vi "XYZ STAGE SERVER.vi"() -> ()   [LabVIEW 2018]
uses:
  STAGE POSITION.ctl
  GOTO POSITION.ctl
  STAGE VELOCITY.ctl
  FIB STAGE EVENTS.ctl
panel:
  in  "OBJECT RANGE":i32(ring) items=["100um", "150um", "200um", "250um", "500um ", "0-1mm Variable", "1mm Aperture", "2mm Aperture", "5mm Aperture", "OPEN"]
  out "VALID SESSION":bool=TRUE
  out "PZ":i32
  out "PY":i32
  out "PX":i32
  in  "ZERO STAGES":bool
  in  "Array":cluster{"POSITION ":T1, "MARKER ID":string}[](array[cluster]) {"POSITION"."Z" format="%_5g"; "POSITION"."Y" format="%_5g"; "POSITION"."X" format="%_5g"}
  out "REPLY":string[](array[string])
  out "COMMAND":string[](array[string])
  out "STAGE ERROR":errorcluster={"status"=FALSE, "code"=1073676293, "source"="VISA Read in ARCUS Object Socket.vi->CSIRO Object Control Ethernet.vi"}
  out "FIB STAGE":refnum<visa-resource-name>="CSIRO-OBJECT"
  out "Z":bool[](array[boolean])=[FALSE, FALSE, FALSE, FALSE, FALSE, FALSE, TRUE, FALSE, FALSE, FALSE, FALSE, FALSE, FALSE, FALSE, FALSE, FALSE]
  out "X":bool[](array[boolean])=[FALSE, FALSE, FALSE, FALSE, FALSE, FALSE, TRUE, FALSE, FALSE, FALSE, FALSE, FALSE, FALSE, FALSE, FALSE, FALSE]
  out "THETA":bool[](array[boolean])=[FALSE, FALSE, FALSE, FALSE, FALSE, FALSE, TRUE, FALSE, FALSE, FALSE, FALSE, FALSE, FALSE, FALSE, FALSE, FALSE]
  out "Y":bool[](array[boolean])=[FALSE, FALSE, FALSE, FALSE, FALSE, FALSE, TRUE, FALSE, FALSE, FALSE, FALSE, FALSE, FALSE, FALSE, FALSE, FALSE]
  in  "RIGHT":bool=TRUE
  in  "LEFT":bool=TRUE
  in  "CLEAR":bool
  out "ERROR OUT":errorcluster
  in  "Tab Control":enum32{"STAGE CONTROL", "VELOCITY/ACC/CAL"}(tab)
  out "POSITION":T1 {"Z" format="%#_5g"; "Y" format="%#_5g"; "X" format="%#_5g"}
  in  "GOTO POSITION":T2 {"Z" format="%#_4g"; "Y" min=-0.019999999552965164 max=0.019999999552965164 step=9.999999747378752e-05 format="%#_5g"; "X" format="%#_5g"}
  out "ZCAL STATUS":bool
  out "YCAL STATUS":bool
  out "XCAL STATUS":bool
  in  "HOME Z":bool
  in  "HOME Y":bool
  in  "HOME X":bool
  in  "XYZ STAGE JOG":T3={"DOWN"=FALSE, "UP"=FALSE, "STEP SIZE"=1, "LEFT"=FALSE, "RIGHT"=FALSE} {"STEP SIZE" items=["1 um", "5 um", "20 um", "50 um", "100 um", "500 um", "2000 um"]}
  in  "ABORT":bool
  in  "STOP":bool
  out "CONTROLLER IP":string="10.100.12.76"
  in  "STAGE VELOCITIES":T4={"X VEL"=0.0020000000949949026, "Y VEL"=0.0020000000949949026, "Z VEL"=0.0010000000474974513} {"X VEL" format="%_2f"}
  in  "STAGE ACCELERATION":T5={"X VEL"=0.05, "Y VEL"=0.05, "Z VEL"=0.0010000000474974513} {"X VEL" format="%_2f"}
  in  "YA":dbl[unit]=2.55e-10 format="%#_5g"
  in  "YB":dbl[unit]=0.000128 format="%#_5g"
  in  "XA":dbl[unit]=2.55e-10 format="%#_5g"
  in  "XB":dbl[unit]=0.000125 format="%#_5g"
  in  "ZA":dbl[unit]=2.55e-10 format="%#_5g"
  in  "ZB":dbl[unit]=0.000128 format="%#_5g"
  in  "OYACC":i32=300 min=1 max=5000
  in  "OXACC":i32=300 min=1 max=5000
  in  "OHSPEED":i32=20000 min=1 max=400000 step=1
  in  "OLSPEED":i32=2000 min=100 max=490550
  # "MOTOR ACCE"
  # "MOTOR DECC"
  # "CONST SPEED"
  # "IN ALARM"
  # "LIMIT+ INPUT"
  # "LIMIT- INPUT"
  # "HOME INPUT"
  # "LIMIT+ERROR"
  # "LIMIT- ERROR"
  # "ALARM ERROR"
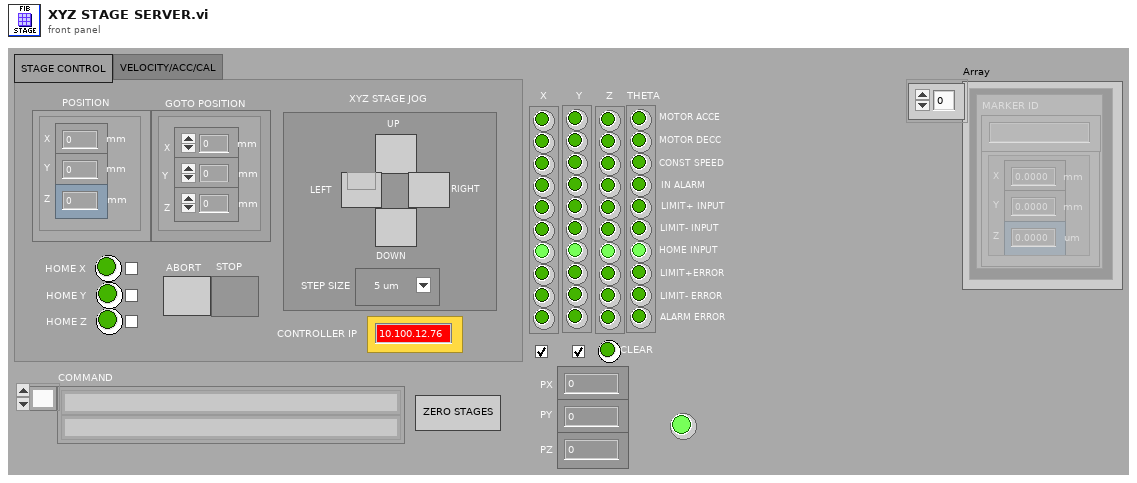
[diagram p1: front panel]
types:
  T1 = typedef "STAGE POSITION.ctl" = cluster{"X":dbl[unit], "Y":dbl[unit], "Z":dbl[unit]}
  T2 = typedef "GOTO POSITION.ctl" = cluster{"X":dbl[unit], "Y":dbl[unit], "Z":dbl[unit]}
  T3 = cluster{"DOWN":bool, "UP":bool, "STEP SIZE":u16, "LEFT":bool, "RIGHT":bool}
  T4 = typedef "STAGE VELOCITY.ctl" = cluster{"X VEL":dbl[unit], "Y VEL":dbl[unit], "Z VEL":dbl[unit]}
  T5 = cluster{"X VEL":dbl[unit], "Y VEL":dbl[unit], "Z VEL":dbl[unit]}
  T6 = typedef "FIB STAGE EVENTS.ctl" = enum16{"LOOP", "INIT STAGE CONTROLLER", "SEND COMMAND TO CONTROLLER", "HOME X", "HOME Y", "HOME Z", "ABORT ALL AXES", "GOTO MARKER", "ZERO XYZ", "READ XYZ POSITIONS", "GOTO XYZ POSITION", "STOP", "JOG XYZ", "WAIT FOR MOVE COMPLETE"}
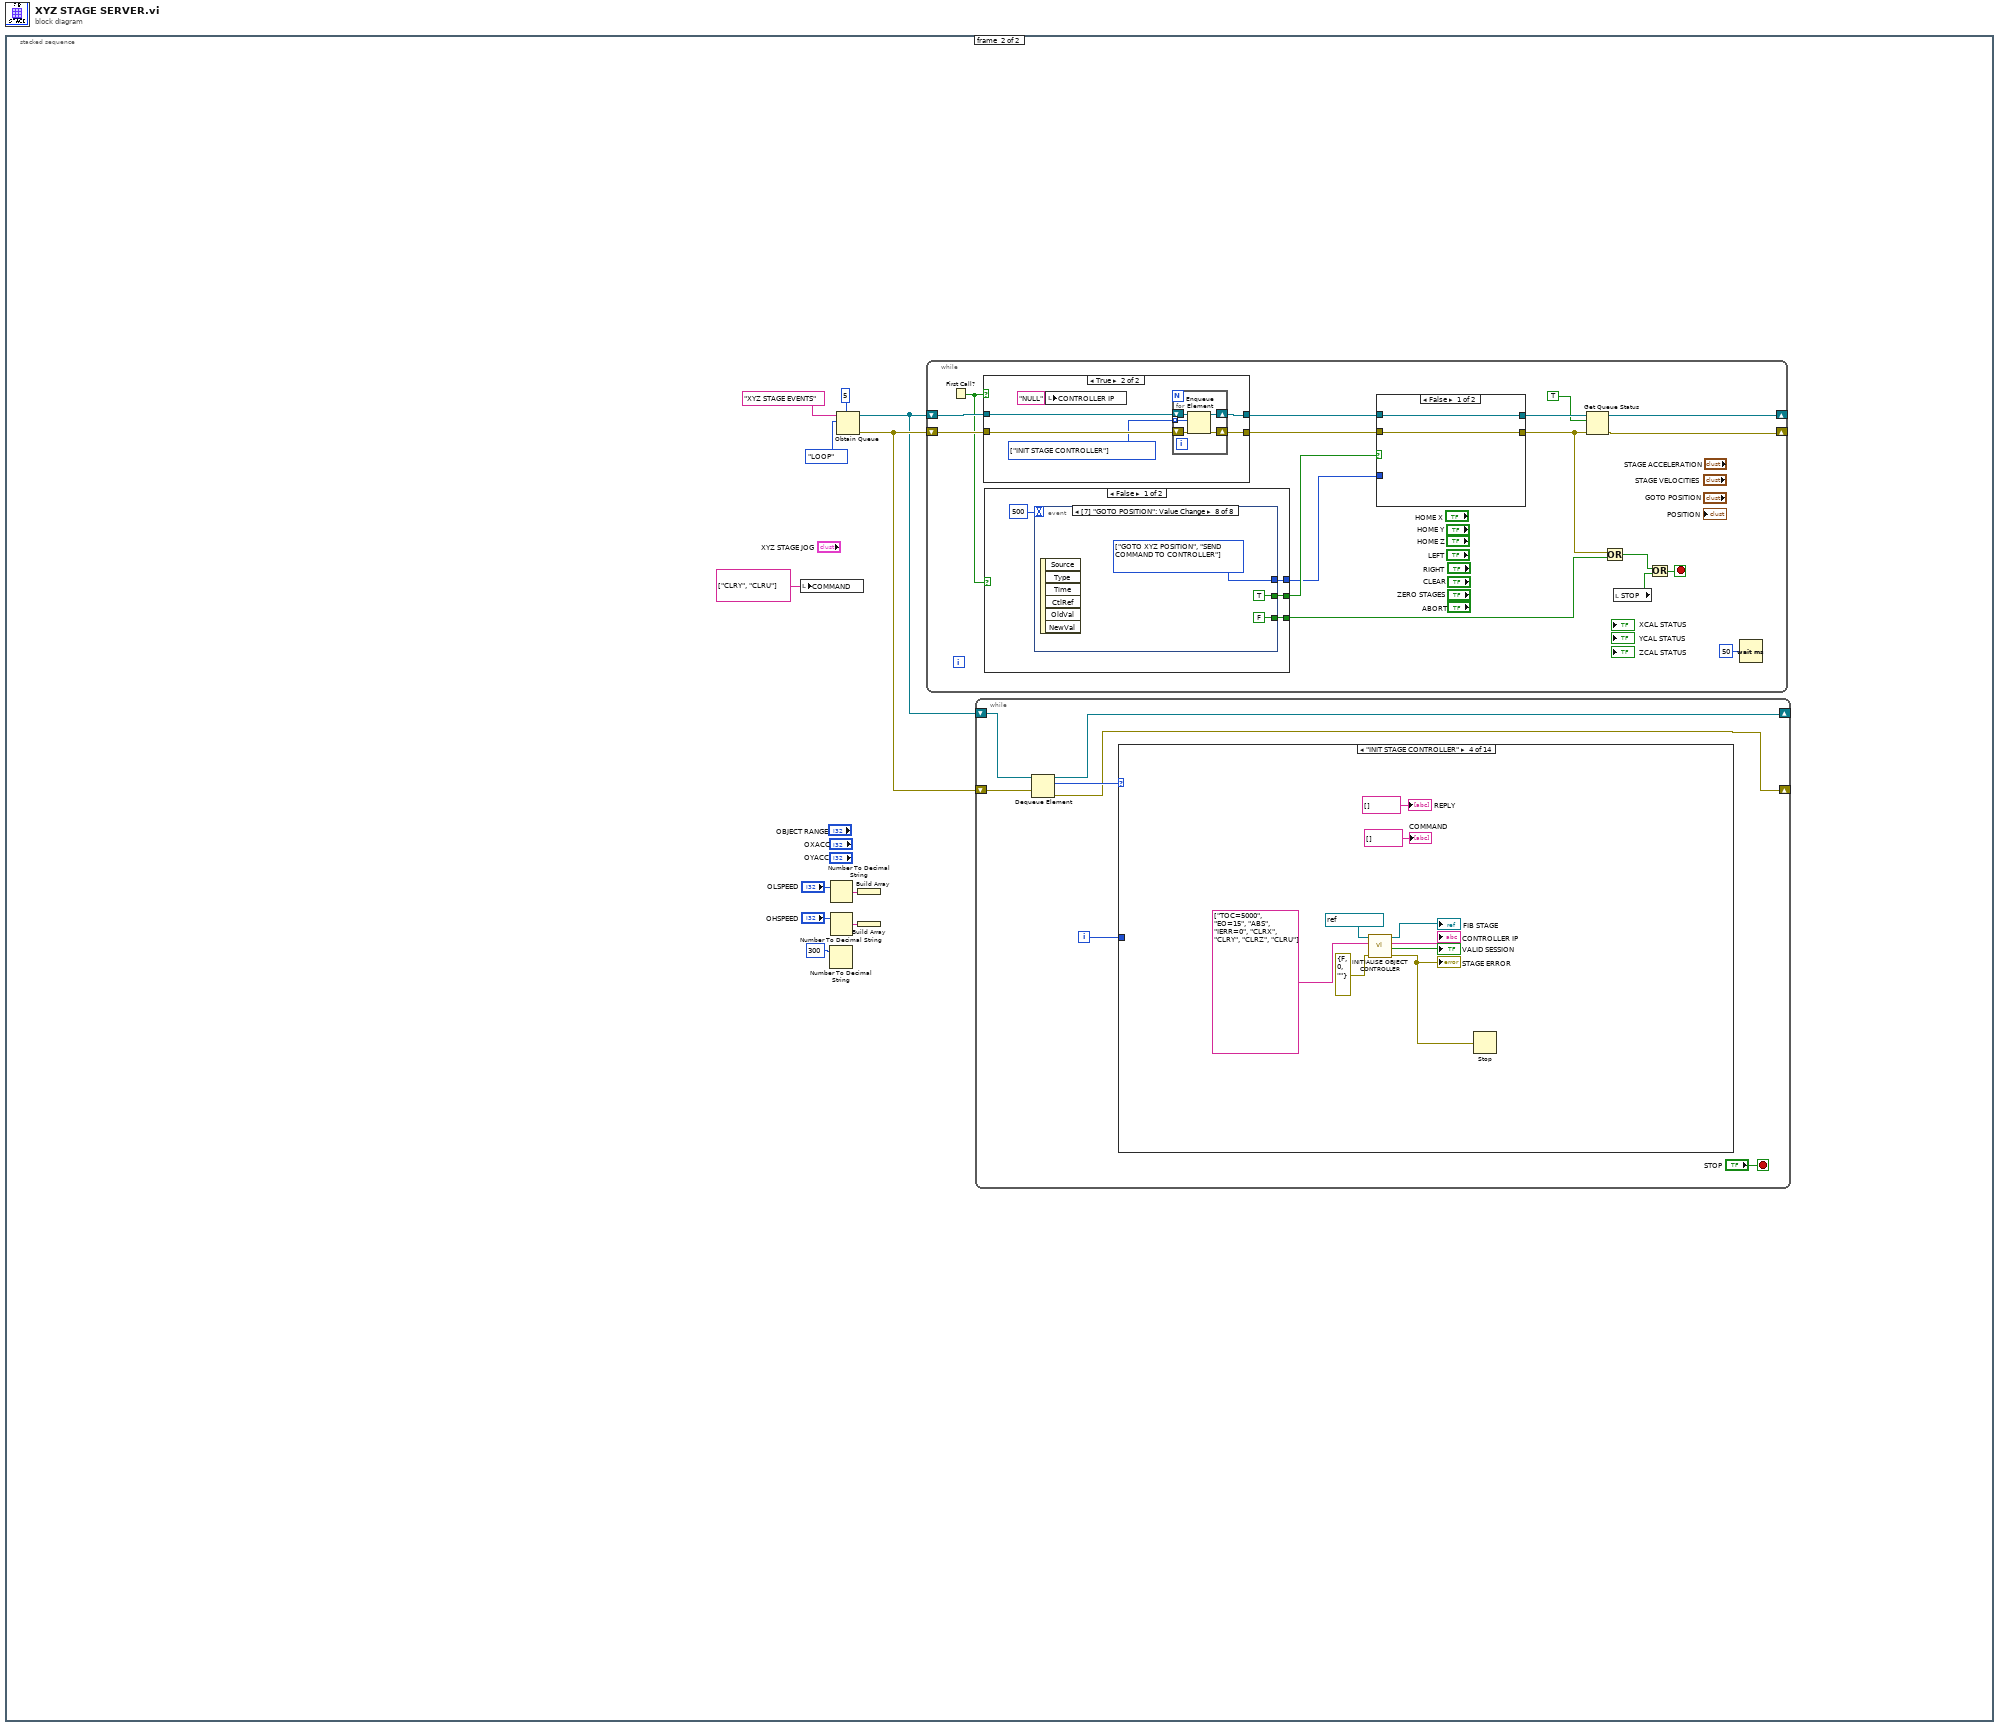
[diagram p0: block diagram]
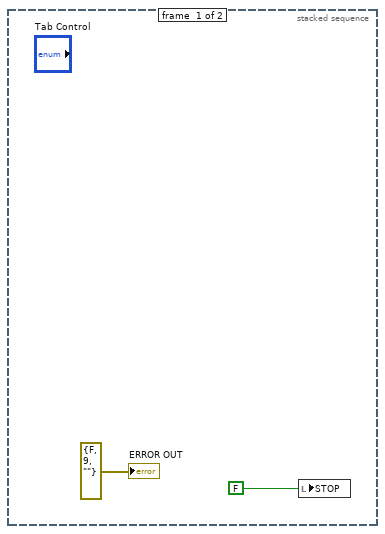
[diagram p2: hidden frame]
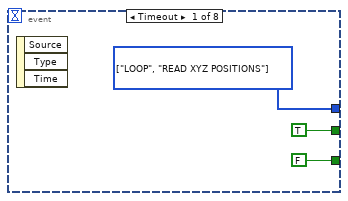
[diagram p3: hidden frame]
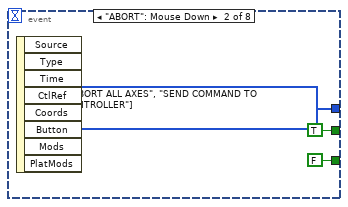
[diagram p4: hidden frame]
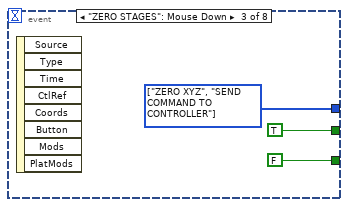
[diagram p5: hidden frame]
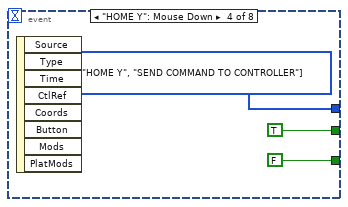
[diagram p6: hidden frame]
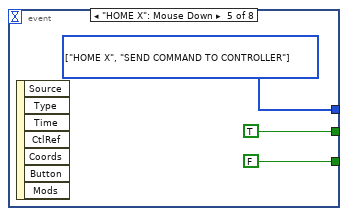
[diagram p7: hidden frame]
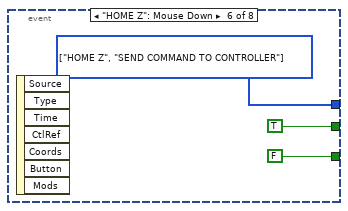
[diagram p8: hidden frame]
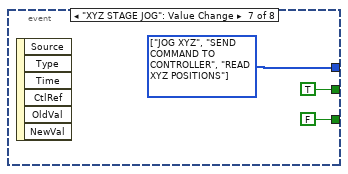
[diagram p9: hidden frame]
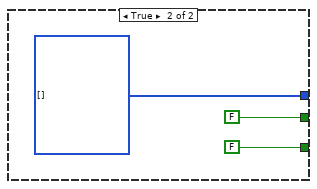
[diagram p10: hidden frame]
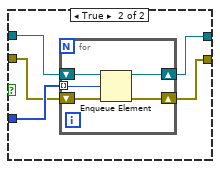
[diagram p11: hidden frame]
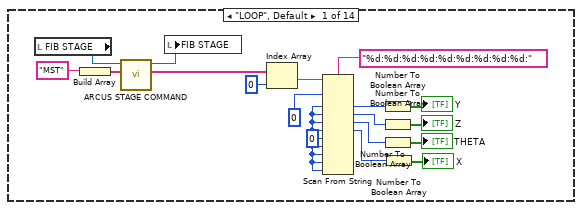
[diagram p13: hidden frame]
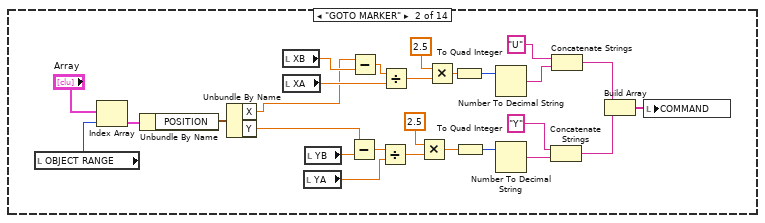
[diagram p14: hidden frame]
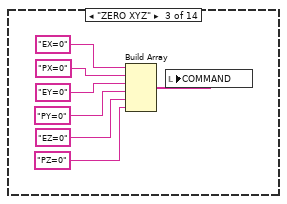
[diagram p15: hidden frame]
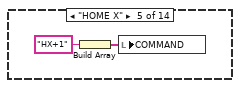
[diagram p16: hidden frame]
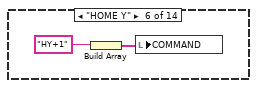
[diagram p17: hidden frame]
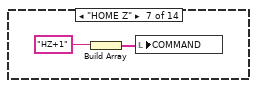
[diagram p18: hidden frame]
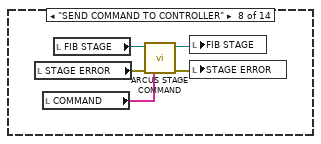
[diagram p19: hidden frame]
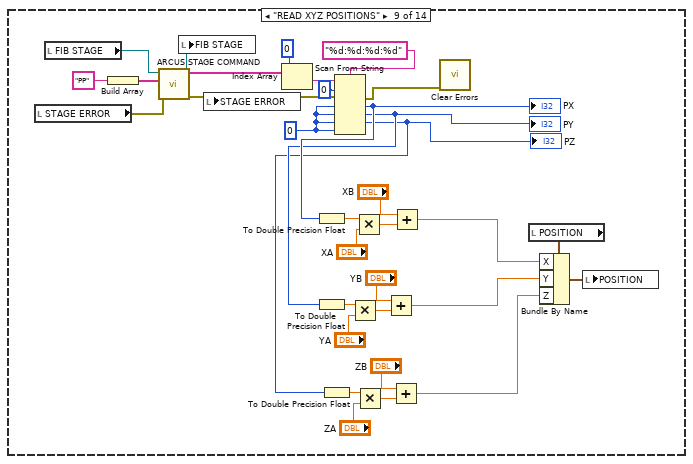
[diagram p20: hidden frame]
diagram:
  n1 = stacked-sequence {
    frame #0 {
      n2 = local write "STOP"(FALSE ("STOP")) -> ()
      "ERROR OUT" <- errorcluster {"status"=FALSE, "code"=9, "source"=""} ("ERROR OUT")
    }
    frame #1 {
      n3 = local write "COMMAND"(string[] ["CLRY", "CLRU"]) -> ()
      n4 = Number To Decimal String(number=300) -> ()  [unwired: 1 in, 1 out]
      n5 = Number To Decimal String(number="OLSPEED") -> (decimal integer string=w8:string)  [unwired: 1 in]
      n6 = Number To Decimal String(number="OHSPEED") -> (decimal integer string=w7:string)  [unwired: 1 in]
      n7 = Obtain Queue(max queue size (-1, unlimited)=5, name (unnamed)="XYZ STAGE EVENTS", element data type=FIB_STAGE_EVENTS."LOOP") -> (queue out=w9:refnum<queue>, error out=w11:errorcluster)  [unwired: 2 in, 1 out]
      n8 = Build Array(w8) -> ()  [unwired: 1 out]
      n9 = Build Array(w7) -> ()  [unwired: 1 out]
      n10 = while {
        shift-right: [w17] -> _
        shift-left: w9 -> [w29]
        shift-right: [w15] -> _
        shift-left: w11 -> [w28]
        stop <- w22 stop-if-true
        n11 = First Call?() -> (First Call?: T/F=w19:bool)
        n12 = case shown="True" w19 {
          tunnel: w29 -> [w75 w81]
          tunnel: w28 -> [w74 w80]
          tunnel: [w75 w79] -> w27
          tunnel: [w74 w78] -> w24
          frame False {
          }
          frame True {
            w77 = T6[] [enum."INIT STAGE CONTROLLER"] items=["LOOP", "INIT STAGE CONTROLLER", "SEND COMMAND TO CONTROLLER", "HOME X", "HOME Y", "HOME Z", "ABORT ALL AXES", "GOTO MARKER", "ZERO XYZ", "READ XYZ POSITIONS", "GOTO XYZ POSITION", "STOP", "JOG XYZ", "WAIT FOR MOVE COMPLETE"]
            n13 = local write "CONTROLLER IP"("NULL" ("CONTROLLER IP")) -> ()
            n14 = for {
              shift-right: [w84] -> w79
              shift-left: w81 -> [w86]
              shift-right: [w83] -> w78
              shift-left: w80 -> [w85]
              tunnel: w77 -> [w82] mode=indexing
              n15 = Enqueue Element(queue=w86, element=w82, error in (no error)=w85) -> (queue out=w84:refnum<queue>, error out=w83:errorcluster)  [unwired: 1 in, 1 out]
            }
          }
        }
        n16 = case shown="False" w19 {
          tunnel: [w33 FALSE] -> w26
          tunnel: [w32 w61] -> w25
          tunnel: [w31 FALSE] -> w21
          frame False {
            n17 = event shown="[7] \"GOTO POSITION\": Value Change" {
              selector: _ -> [_ _ _ _ _ _ _ _]
              dyn-events: _ -> [_ _ _ _ _ _ _ _]
              timeout: 500 -> [_ _ _ _ _ _ _ _]
              tunnel: [TRUE TRUE TRUE TRUE TRUE TRUE TRUE TRUE] -> w33
              tunnel: [FALSE FALSE FALSE FALSE FALSE FALSE FALSE FALSE] -> w31
              tunnel: [w37 w40 w43 w46 w47 w52 w55 w58] -> w32
              event Timeout {
                w37 = T6[] [enum."LOOP", enum."READ XYZ POSITIONS"] items=["LOOP", "INIT STAGE CONTROLLER", "SEND COMMAND TO CONTROLLER", "HOME X", "HOME Y", "HOME Z", "ABORT ALL AXES", "GOTO MARKER", "ZERO XYZ", "READ XYZ POSITIONS", "GOTO XYZ POSITION", "STOP", "JOG XYZ", "WAIT FOR MOVE COMPLETE"]
                n18 = event-data() -> ()  [unwired: 1 in, 3 out]
              }
              event "ABORT": Mouse Down {
                w40 = T6[] [enum."ABORT ALL AXES", enum."SEND COMMAND TO CONTROLLER"] items=["LOOP", "INIT STAGE CONTROLLER", "SEND COMMAND TO CONTROLLER", "HOME X", "HOME Y", "HOME Z", "ABORT ALL AXES", "GOTO MARKER", "ZERO XYZ", "READ XYZ POSITIONS", "GOTO XYZ POSITION", "STOP", "JOG XYZ", "WAIT FOR MOVE COMPLETE"]
                n19 = event-data() -> ()  [unwired: 1 in, 8 out]
              }
              event "ZERO STAGES": Mouse Down {
                w43 = T6[] [enum."ZERO XYZ", enum."SEND COMMAND TO CONTROLLER"] items=["LOOP", "INIT STAGE CONTROLLER", "SEND COMMAND TO CONTROLLER", "HOME X", "HOME Y", "HOME Z", "ABORT ALL AXES", "GOTO MARKER", "ZERO XYZ", "READ XYZ POSITIONS", "GOTO XYZ POSITION", "STOP", "JOG XYZ", "WAIT FOR MOVE COMPLETE"]
                n20 = event-data() -> ()  [unwired: 1 in, 8 out]
              }
              event "HOME Y": Mouse Down {
                w46 = T6[] [enum."HOME Y", enum."SEND COMMAND TO CONTROLLER"] items=["LOOP", "INIT STAGE CONTROLLER", "SEND COMMAND TO CONTROLLER", "HOME X", "HOME Y", "HOME Z", "ABORT ALL AXES", "GOTO MARKER", "ZERO XYZ", "READ XYZ POSITIONS", "GOTO XYZ POSITION", "STOP", "JOG XYZ", "WAIT FOR MOVE COMPLETE"]
                n21 = event-data() -> ()  [unwired: 1 in, 8 out]
              }
              event "HOME X": Mouse Down {
                w47 = T6[] [enum."HOME X", enum."SEND COMMAND TO CONTROLLER"] items=["LOOP", "INIT STAGE CONTROLLER", "SEND COMMAND TO CONTROLLER", "HOME X", "HOME Y", "HOME Z", "ABORT ALL AXES", "GOTO MARKER", "ZERO XYZ", "READ XYZ POSITIONS", "GOTO XYZ POSITION", "STOP", "JOG XYZ", "WAIT FOR MOVE COMPLETE"]
                n22 = event-data() -> ()  [unwired: 1 in, 7 out]
              }
              event "HOME Z": Mouse Down {
                w52 = T6[] [enum."HOME Z", enum."SEND COMMAND TO CONTROLLER"] items=["LOOP", "INIT STAGE CONTROLLER", "SEND COMMAND TO CONTROLLER", "HOME X", "HOME Y", "HOME Z", "ABORT ALL AXES", "GOTO MARKER", "ZERO XYZ", "READ XYZ POSITIONS", "GOTO XYZ POSITION", "STOP", "JOG XYZ", "WAIT FOR MOVE COMPLETE"]
                n23 = event-data() -> ()  [unwired: 1 in, 7 out]
              }
              event "XYZ STAGE JOG": Value Change {
                w55 = T6[] [enum."JOG XYZ", enum."SEND COMMAND TO CONTROLLER", enum."READ XYZ POSITIONS"] items=["LOOP", "INIT STAGE CONTROLLER", "SEND COMMAND TO CONTROLLER", "HOME X", "HOME Y", "HOME Z", "ABORT ALL AXES", "GOTO MARKER", "ZERO XYZ", "READ XYZ POSITIONS", "GOTO XYZ POSITION", "STOP", "JOG XYZ", "WAIT FOR MOVE COMPLETE"]
                n24 = event-data() -> ()  [unwired: 1 in, 6 out]
              }
              event Value Change {
                w58 = T6[] [enum."GOTO XYZ POSITION", enum."SEND COMMAND TO CONTROLLER"] items=["LOOP", "INIT STAGE CONTROLLER", "SEND COMMAND TO CONTROLLER", "HOME X", "HOME Y", "HOME Z", "ABORT ALL AXES", "GOTO MARKER", "ZERO XYZ", "READ XYZ POSITIONS", "GOTO XYZ POSITION", "STOP", "JOG XYZ", "WAIT FOR MOVE COMPLETE"]
                n25 = event-data() -> ()  [unwired: 1 in, 6 out]
              }
            }
          }
          frame True {
            w61 = T6[] [] items=["LOOP", "INIT STAGE CONTROLLER", "SEND COMMAND TO CONTROLLER", "HOME X", "HOME Y", "HOME Z", "ABORT ALL AXES", "GOTO MARKER", "ZERO XYZ", "READ XYZ POSITIONS", "GOTO XYZ POSITION", "STOP", "JOG XYZ", "WAIT FOR MOVE COMPLETE"]
          }
        }
        n26 = case shown="False" w26 {
          tunnel: w27 -> [w63 w68]
          tunnel: w25 -> [_ w67]
          tunnel: [w63 w66] -> w18
          tunnel: [w62 w65] -> w16
          tunnel: w24 -> [w62 w64]
          frame False {
          }
          frame True {
            n27 = for {
              shift-right: [w71] -> w66
              shift-left: w68 -> [w73]
              shift-right: [w70] -> w65
              shift-left: w64 -> [w72]
              tunnel: w67 -> [w69] mode=indexing
              n28 = Enqueue Element(queue=w73, element=w69, error in (no error)=w72) -> (queue out=w71:refnum<queue>, error out=w70:errorcluster)  [unwired: 1 in, 1 out]
            }
          }
        }
        n29 = Get Queue Status(queue=w18, return elements? (F)=TRUE, error in (no error)=w16) -> (queue out=w17:refnum<queue>, error out=w15:errorcluster)  [unwired: 6 out]
        n30 = Or(x=w16, y=w21) -> (x .or. y?=w20:bool)
        n31 = local read "STOP"() -> (w23:bool)
        n32 = Or(x=w20, y=w23) -> (x .or. y?=w22:bool)
        n33 = Wait (ms)(milliseconds to wait=u32 50) -> ()  [unwired: 1 out]
      }
      n34 = while {
        shift-right: [w88] -> _
        shift-left: w9 -> [w90]
        shift-right: [w87] -> _
        shift-left: w11 -> [w92]
        i -> [w89]
        stop <- "STOP" stop-if-true
        n35 = Dequeue Element(queue=w90, error in (no error)=w92) -> (queue out=w88:refnum<queue>, element=w91:T6, error out=w87:errorcluster)  [unwired: 1 in, 1 out]
        n36 = case shown="\"INIT STAGE CONTROLLER\"" w91 {
          tunnel: w89 -> [_ _ _ _ _ _ _ _ _ _ _ _ _ _]
          frame "LOOP", Default {
            w96 = u16 0 ("default value 5")
            n37 = local read "FIB STAGE"() -> (w95:refnum<visa-resource-name>)
            n38 = Build Array("MST" ("write_string")) -> (w105:string[])
            n39 = call "ARCUS STAGE COMMAND.vi"("COMMANDS"=w105, "OBJECT IN"=w95) -> ("OUTPUT"=w104:string[], "OBJECT OUT"=w94:refnum<visa-resource-name>)  [unwired: 7 in, 1 out]
            n40 = local write "FIB STAGE"(w94) -> ()
            n41 = Index Array(array=w104, index=0) -> (element=w103:string)
            n42 = Scan From String(format string="%d:%d:%d:%d:%d:%d:%d:%d:%d:", input string=w103, initial scan location=u32 0, default 1=w96, default 2=w96, default 3=w96, default 4=w96, default 5=w96, default 6=w96, default 7=w96, default 8=w96, default 9=w96) -> (output 1=w111:u16, output 2=w110:u16, output 3=w109:u16, output 4=w108:u16)  [unwired: 6 in, 3 out]
            n43 = Number To Boolean Array(number=w111) -> (Boolean array=→"Y":bool[])
            n44 = Number To Boolean Array(number=w110) -> (Boolean array=→"Z":bool[])
            n45 = Number To Boolean Array(number=w109) -> (Boolean array=→"THETA":bool[])
            n46 = Number To Boolean Array(number=w108) -> (Boolean array=→"X":bool[])
          }
          frame "GOTO MARKER" {
            n47 = local read "OBJECT RANGE"() -> (w138:i32)
            n48 = Index Array(array="Array", index=w138) -> (element=w120:cluster{"POSITION ":T1, "MARKER ID":string})
            n49 = Unbundle By Name(w120) -> ("POSITION"=w114:T1)
            n50 = Unbundle By Name(w114) -> ("X"=w113:dbl[unit], "Y"=w112:dbl[unit])
            n51 = local read "XB"() -> (w136:dbl[unit])
            n52 = local read "XA"() -> (w134:dbl[unit])
            n53 = local read "YA"() -> (w131:dbl[unit])
            n54 = local read "YB"() -> (w132:dbl[unit])
            n55 = Subtract(x=w112, y=w132) -> (x-y=w133:dbl[unit])
            n56 = Subtract(x=w113, y=w136) -> (x-y=w135:dbl[unit])
            n57 = Divide(x=w133, y=w131) -> (x/y=w122:dbl)
            n58 = Divide(x=w135, y=w134) -> (x/y=w124:dbl)
            n59 = Multiply(x=sgl 2.5, y=w122) -> (x*y=w123:dbl)
            n60 = Multiply(x=sgl 2.5, y=w124) -> (x*y=w125:dbl)
            n61 = To Quad Integer(1:w125) -> (0:w126:i64)
            n62 = To Quad Integer(1:w123) -> (0:w121:i64)
            n63 = Number To Decimal String(number=w126) -> (decimal integer string=w129:string)  [unwired: 1 out]
            n64 = Number To Decimal String(number=w121) -> (decimal integer string=w128:string)  [unwired: 1 out]
            n65 = Concatenate Strings("Y", w128) -> (w127:string)
            n66 = Concatenate Strings("U", w129) -> (w130:string)
            n67 = Build Array(w130, w127) -> (w137:string[])
            n68 = local write "COMMAND"(w137) -> ()
          }
          frame "ZERO XYZ" {
            n69 = Build Array("EX=0" ("write_string"), "PX=0" ("write_string"), "EY=0" ("write_string"), "PY=0" ("write_string"), "EZ=0" ("write_string"), "PZ=0" ("write_string")) -> (w145:string[])
            n70 = local write "COMMAND"(w145) -> ()
          }
          frame "INIT STAGE CONTROLLER" {
            n71 = call "INITIALISE OBJECT CONTROLLER.vi"("error in (no error)"=errorcluster {"status"=FALSE, "code"=0, "source"=""}, "INIITIALISE"=string[] ["TOC=5000", "EO=15", "ABS", "IERR=0", "CLRX", "CLRY", "CLRZ", "CLRU"], "FIB STAGE"=refnum<visa-resource-name> "FIBSTAGE" ("VISA resource name")) -> ("ERROR OUT"=w146:errorcluster, "VALID SESSION"=→"VALID SESSION":bool, "TCP/IP Settings:Dot-Notation Address"=→"CONTROLLER IP":string, "FIB STAGE"=→"FIB STAGE":refnum<visa-resource-name>)  [unwired: 4 in, 1 out]
            "STAGE ERROR" <- w146
            n72 = Stop(stop? (T)=w146) -> ()
            "COMMAND" <- string[] [] ("COMMAND")
            "REPLY" <- string[] [] ("REPLY")
          }
          frame "HOME X" {
            n73 = Build Array("HX+1" ("COMMAND")) -> (w156:string[])
            n74 = local write "COMMAND"(w156) -> ()
          }
          frame "HOME Y" {
            n75 = Build Array("HY+1" ("COMMAND")) -> (w158:string[])
            n76 = local write "COMMAND"(w158) -> ()
          }
          frame "HOME Z" {
            n77 = Build Array("HZ+1" ("COMMAND")) -> (w160:string[])
            n78 = local write "COMMAND"(w160) -> ()
          }
          frame "SEND COMMAND TO CONTROLLER" {
            n79 = local read "STAGE ERROR"() -> (w163:errorcluster)
            n80 = local read "COMMAND"() -> (w161:string[])
            n81 = local read "FIB STAGE"() -> (w162:refnum<visa-resource-name>)
            n82 = call "ARCUS STAGE COMMAND.vi"("error in (no error)"=w163, "COMMANDS"=w161, "OBJECT IN"=w162) -> ("error out"=w164:errorcluster, "OBJECT OUT"=w165:refnum<visa-resource-name>)  [unwired: 6 in, 1 out]
            n83 = local write "FIB STAGE"(w165) -> ()
            n84 = local write "STAGE ERROR"(w164) -> ()
          }
          frame "READ XYZ POSITIONS" {
            w192 = 0 ("default value 5")
            n85 = local read "STAGE ERROR"() -> (w189:errorcluster)
            n86 = local read "FIB STAGE"() -> (w188:refnum<visa-resource-name>)
            n87 = Build Array("PP" ("write_string")) -> (w195:string[])
            n88 = call "ARCUS STAGE COMMAND.vi"("error in (no error)"=w189, "COMMANDS"=w195, "OBJECT IN"=w188) -> ("error out"=w186:errorcluster, "OUTPUT"=w196:string[], "OBJECT OUT"=w187:refnum<visa-resource-name>)  [unwired: 6 in]
            n89 = local write "FIB STAGE"(w187) -> ()
            n90 = local write "STAGE ERROR"(w186) -> ()
            n91 = Index Array(array=w196, index=0) -> (element=w197:string)
            n92 = Scan From String(format string="%d:%d:%d:%d", input string=w197, initial scan location=u32 0, error in=w186, default 1=w192, default 2=w192, default 3=w192, default 4=w192) -> (error out=w198:errorcluster, output 1=w177:i32, output 2=w167:i32, output 3=w166:i32)  [unwired: 1 in, 2 out]
            "PX" <- w177
            "PY" <- w167
            "PZ" <- w166
            n93 = To Double Precision Float(number=w177) -> (double precision float=w178:dbl)
            n94 = To Double Precision Float(number=w167) -> (double precision float=w183:dbl)
            n95 = To Double Precision Float(number=w166) -> (double precision float=w170:dbl)
            n96 = Multiply(x=w183, y="YA") -> (x*y=w184:dbl[unit])
            n97 = Multiply(x=w178, y="XA") -> (x*y=w180:dbl[unit])
            n98 = Multiply(x=w170, y="ZA") -> (x*y=w171:dbl[unit])
            n99 = Add(x="YB", y=w184) -> (x+y=w173:dbl[unit])
            n100 = Add(x="ZB", y=w171) -> (x+y=w168:dbl[unit])
            n101 = Add(x="XB", y=w180) -> (x+y=w174:dbl[unit])
            n102 = call <vilib>:"Clear Errors.vi"("error in (no error)"=w198) -> ()  [unwired: 5 in, 2 out]
            n103 = local read "POSITION"() -> (w175:T1)
            n104 = Bundle By Name(cluster=w175, "X"=w174, "Y"=w173, "Z"=w168) -> (w176:T1)
            n105 = local write "POSITION"(w176) -> ()
          }
          frame "GOTO XYZ POSITION" {
            n106 = local read "GOTO POSITION"() -> (w225:T2)
            n107 = Unbundle By Name(w225) -> ("X"=w224:dbl[unit], "Y"=w204:dbl[unit], "Z"=w201:dbl[unit])
            n108 = local read "XB"() -> (w223:dbl[unit])
            n109 = local read "YB"() -> (w203:dbl[unit])
            n110 = local read "ZB"() -> (w200:dbl[unit])
            n111 = local read "XA"() -> (w221:dbl[unit])
            n112 = local read "ZA"() -> (w199:dbl[unit])
            n113 = local read "YA"() -> (w202:dbl[unit])
            n114 = Subtract(x=w201, y=w200) -> (x-y=w213:dbl[unit])
            n115 = Subtract(x=w224, y=w223) -> (x-y=w222:dbl[unit])
            n116 = Subtract(x=w204, y=w203) -> (x-y=w216:dbl[unit])
            n117 = Divide(x=w213, y=w199) -> (x/y=w212:dbl)
            n118 = Divide(x=w222, y=w221) -> (x/y=w220:dbl)
            n119 = Divide(x=w216, y=w202) -> (x/y=w215:dbl)
            n120 = To Long Integer(number=w212) -> (32bit integer=w211:i32)
            n121 = To Long Integer(number=w220) -> (32bit integer=w219:i32)
            n122 = To Long Integer(number=w215) -> (32bit integer=w214:i32)
            n123 = Number To Decimal String(number=w211) -> (decimal integer string=w208:string)  [unwired: 1 in]
            n124 = Number To Decimal String(number=w219) -> (decimal integer string=w217:string)  [unwired: 1 in]
            n125 = Number To Decimal String(number=w214) -> (decimal integer string=w209:string)  [unwired: 1 in]
            n126 = Concatenate Strings("X" ("string"), w217, "Y" ("string"), w209, "Z" ("string"), w208) -> (w206:string)
            n127 = Build Array(w206) -> (w205:string[])
            n128 = local write "COMMAND"(w205) -> ()
          }
          frame "WAIT FOR MOVE COMPLETE" {
          }
          frame "STOP" {
          }
          frame "JOG XYZ" {
            n129 = local read "XYZ STAGE JOG"() -> (w237:T3)
            n130 = Unbundle By Name(w237) -> ("UP"=w236:bool, "DOWN"=w235:bool, "LEFT"=w234:bool, "RIGHT"=w233:bool, "STEP SIZE"=w230:u16)
            n131 = case shown="1" w230 {
              tunnel: [1000 2000] -> w229
              frame 0, Default {
              }
              frame 1 {
              }
            }
            n132 = Build Array(w236, w235, w234, w233) -> (w232:bool[])
            n133 = local read "PX"() -> (w226:i32)
            n134 = local read "PY"() -> (w227:i32)
            n135 = Boolean Array To Number(Boolean array=w232) -> (number=w231:u32)
            n136 = case shown="0, Default" w231 {
              tunnel: w229 -> [_ w245 w251 w257 w264]
              tunnel: [w241 w243 w250 w258 w265] -> w228
              tunnel: w227 -> [_ w242 w249 _ _]
              tunnel: w226 -> [_ _ _ w256 w263]
              frame 0, Default {
                n137 = Build Array("STOP") -> (w241:string[])
              }
              frame 1 {
                n138 = Add(x=w242, y=w245) -> (x+y=w244:i32)
                n139 = Number To Decimal String(number=w244) -> (decimal integer string=w248:string)  [unwired: 1 in]
                n140 = Concatenate Strings("Y", w248) -> (w247:string)
                n141 = Build Array(w247) -> (w243:string[])
              }
              frame 2 {
                n142 = Subtract(x=w249, y=w251) -> (x-y=w252:i32)
                n143 = Number To Decimal String(number=w252) -> (decimal integer string=w255:string)  [unwired: 1 in]
                n144 = Concatenate Strings("Y", w255) -> (w254:string)
                n145 = Build Array(w254) -> (w250:string[])
              }
              frame 4 {
                n146 = Subtract(x=w256, y=w257) -> (x-y=w259:i32)
                n147 = Number To Decimal String(number=w259) -> (decimal integer string=w262:string)  [unwired: 1 in]
                n148 = Concatenate Strings("X", w262) -> (w261:string)
                n149 = Build Array(w261) -> (w258:string[])
              }
              frame 8 {
                n150 = Add(x=w263, y=w264) -> (x+y=w266:i32)
                n151 = Number To Decimal String(number=w266) -> (decimal integer string=w269:string)  [unwired: 1 in]
                n152 = Concatenate Strings("X", w269) -> (w268:string)
                n153 = Build Array(w268) -> (w265:string[])
              }
            }
            n154 = local write "COMMAND"(w228) -> ()
          }
          frame "ABORT ALL AXES" {
            n155 = local write "COMMAND"(string[] ["ABORT"]) -> ()
          }
        }
      }
    }
  }
